vi "Renishaw-XL80_GetDX10Status.vi"(8 "error in (no error)":errorcluster, 11 "Renishaw-XL80 in":refnum<class "Renishaw-XL80.lvclass">) -> (0 "error out":errorcluster, 2 "DX10Status":i32(ring) items=["DX10_CONNECTED", "DX10_NOT_RESPONDING"], 3 "Renishaw-XL80 out":refnum<class "Renishaw-XL80.lvclass">)   [LabVIEW 2024, in "Renishaw-XL80.lvclass"]
doc: "DX10Status property\nThis read only property returns the current status of the DX10. It indicates whether or not the DX10 is responding.\n\nDefinition\nHRESULT\nget_DX10Status(\n [out, retval] DX10_STATUS_CODES* pVal\n);\n\nParameters\npVal\nA variable that will be set one of the DX10_STATUS_CODES.\n\nComments\nThis property will return with an HRESULT of E_FAIL if the client has not previously connected to a DX10 by calling Connect.\n\nThe property will normally return an HRESULT of S_OK. However, it will return E_POINTER if the client supplies a null pointer for pVal.\n\nNote: if there is a XL laser connected to the DX10Adaptor COM interface this property relates to a virtual DX10 and will always return DX10_CONNECTED."
uses:
  Renishaw-XL80.lvclass
  Renishaw-XL80.lvclass/Renishaw-XL80.ctl
  D:/A.C.M/Example CSharp_64/bin/Debug/Interop.DX10SDKADAPTORLib.dll
  Example CSharp_64/bin/Debug/Interop.DX10SDKADAPTORLib.dll
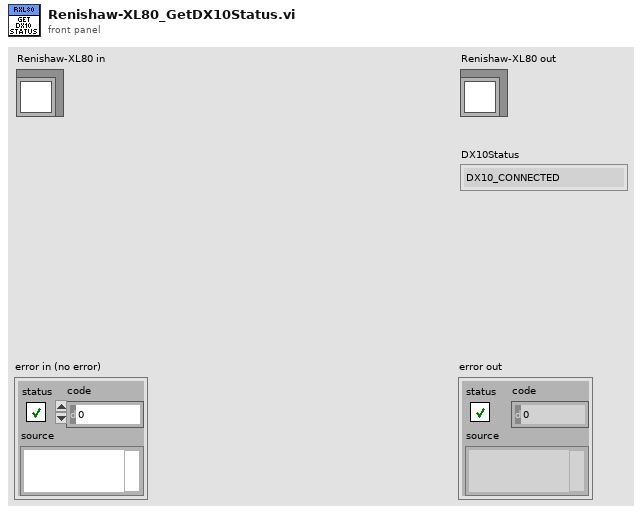
[diagram p1: front panel]
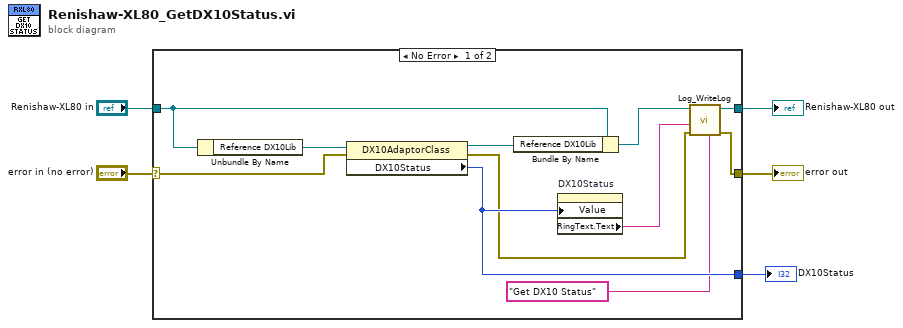
[diagram p0: block diagram]
diagram:
  n1 = case shown="No Error" "error in (no error)" {
    selector: "error in (no error)" -> [w15 w18]
    tunnel: [w8 w18] -> w4
    tunnel: [w11 w17] -> w2
    tunnel: "Renishaw-XL80 in" -> [w14 w17]
    tunnel: [w10 _] -> w1
    frame No Error {
      n2 = Unbundle By Name(w14) -> ("Reference DX10Lib"=w16:refnum<k24>)
      n3 = property class="DX10AdaptorClass"(reference=w16, error in=w15) -> (reference out=w13:refnum<k24>, error out=w6:errorcluster, "DX10Status"=w10:i32)
      n4 = Bundle By Name(cluster=w14, "Reference DX10Lib"=w13) -> (w12:refnum<class "Renishaw-XL80.lvclass">)
      n5 = property on="DX10Status" class="Ring (strict)"("Value"=w10) -> ("RingText.Text"=w9:string)  [unwired: 2 in, 2 out]
      n6 = call-dynamic "Log_WriteLog.vi"("Additional text"="Get DX10 Status", "error in (no error)"=w6, "Response"=w9, "Log in"=w12) -> ("error out"=w8:errorcluster, "Log out"=w11:refnum<class "Renishaw-XL80.lvclass">)  [unwired: 6 in]
    }
    frame Error {
    }
  }
  "error out" <- w4
  "Renishaw-XL80 out" <- w2
  "DX10Status" <- w1
